vi "Address Compute.vi"(10 "address type (DD RAM)":enum16{"DDRAM", "CGRAM"}(ring), 11 "input address":u8 format="%.0x") -> (3 "output address":u8)   [LabVIEW 2015, in "HD44780 Common.lvlib"]
uses:
  HD44780 Common.lvlib
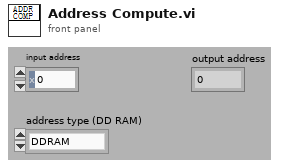
[diagram p1: front panel]
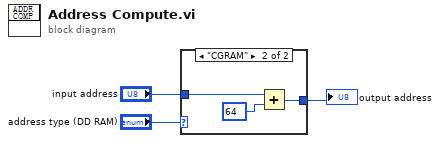
[diagram p0: block diagram]
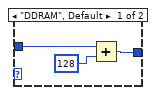
[diagram p2: hidden frame]
diagram:
  n1 = case shown="\"CGRAM\"" "address type (DD RAM)" {
    tunnel: "input address" -> [w5 w8]
    tunnel: [w4 w7] -> w3
    frame "DDRAM", Default {
      n2 = Add(x=w5, y=u8 128) -> (x+y=w4:u8)
    }
    frame "CGRAM" {
      n3 = Add(x=w8, y=u8 64) -> (x+y=w7:u8)
    }
  }
  "output address" <- w3
